vi "PXI-Set Property.vi"(0 "Key":string, 7 "Value":variant, 11 "error in (no error)":errorcluster) -> (15 "error out":errorcluster)   [LabVIEW 2015]
uses:
  DAQ Engine VIs/PXI Globals.vi
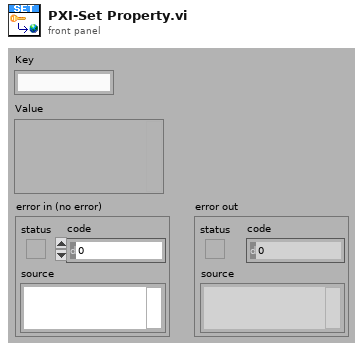
[diagram p1: front panel]
types:
  T1 = typedef "Counter Params.ctl" = cluster{"Counter":tag, "Hi ticks":u32, "Low ticks":u32, "Idle state":i32, "Delay ticks":u32}
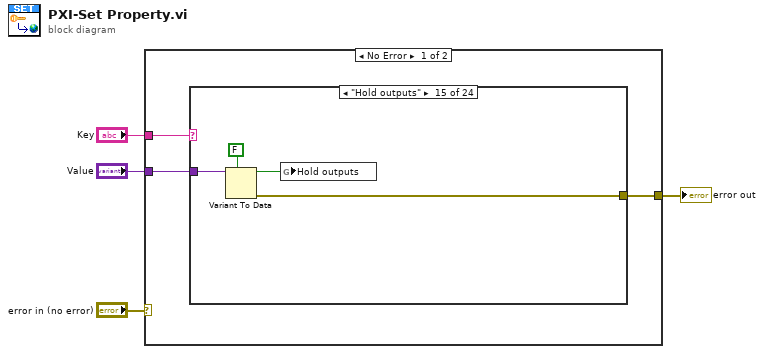
[diagram p0: block diagram]
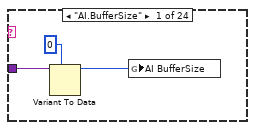
[diagram p2: hidden frame]
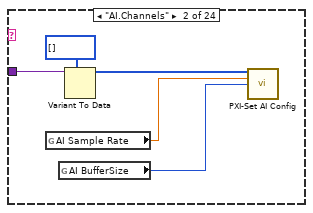
[diagram p3: hidden frame]
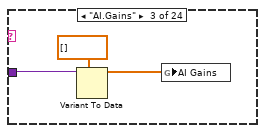
[diagram p4: hidden frame]
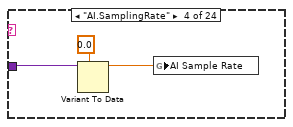
[diagram p5: hidden frame]
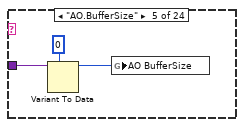
[diagram p6: hidden frame]
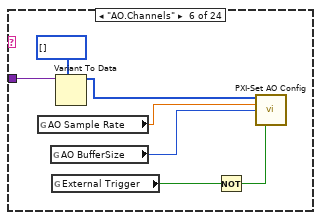
[diagram p7: hidden frame]
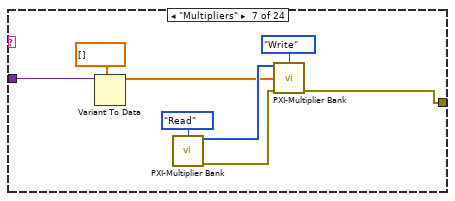
[diagram p8: hidden frame]
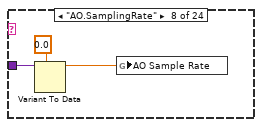
[diagram p9: hidden frame]
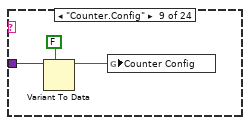
[diagram p10: hidden frame]
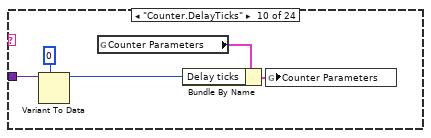
[diagram p11: hidden frame]
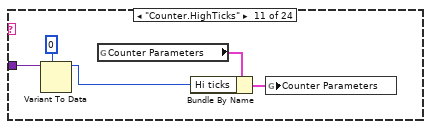
[diagram p12: hidden frame]
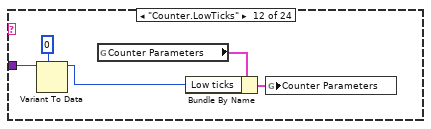
[diagram p13: hidden frame]
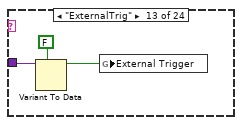
[diagram p14: hidden frame]
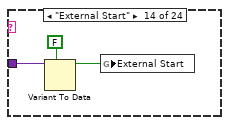
[diagram p15: hidden frame]
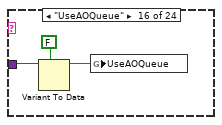
[diagram p16: hidden frame]
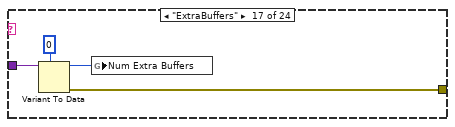
[diagram p17: hidden frame]
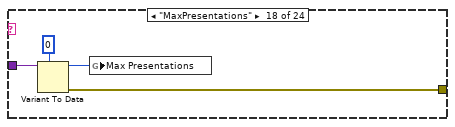
[diagram p18: hidden frame]
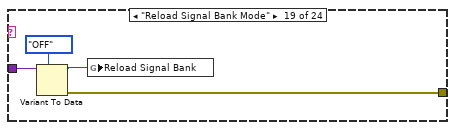
[diagram p19: hidden frame]
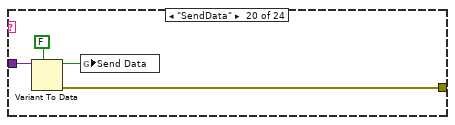
[diagram p20: hidden frame]
diagram:
  n1 = case shown="No Error" "error in (no error)" {
    selector: "error in (no error)" -> [_ w107]
    tunnel: "Key" -> [w7 _]
    tunnel: "Value" -> [w6 _]
    tunnel: [w5 w107] -> w1
    frame No Error {
      n2 = case shown="\"Hold outputs\"" w7 {
        selector: w7 -> [_ _ _ _ _ _ _ _ _ _ _ _ _ _ _ _ _ _ _ _ _ _ _ w104]
        tunnel: w6 -> [w10 w12 w17 w20 w23 w26 w33 w41 w44 w47 w52 w57 w62 w65 w69 w72 w76 w80 w85 w88 w92 w96 w100 _]
        tunnel: [_ _ _ _ _ _ w35 _ _ _ _ _ _ _ w67 _ w74 w78 w82 w86 w90 w94 w98 w102] -> w5
        frame "AI.BufferSize" {
          n3 = Variant To Data(type=0, Variant=w10) -> (data=w8:i32)  [unwired: 1 in, 1 out]
          n4 = global write "PXI Globals.vi" "AI BufferSize"(w8) -> ()
        }
        frame "AI.Channels" {
          n5 = global read "PXI Globals.vi" "AI Sample Rate"() -> (w15:dbl)
          n6 = global read "PXI Globals.vi" "AI BufferSize"() -> (w14:i32)
          n7 = Variant To Data(type=i32[] [], Variant=w12) -> (data=w11:i32[])  [unwired: 1 in, 1 out]
          n8 = call "PXI-Set AI Config.vi"("AI Channels"=w11, "Sampling Rate (Hz)"=w15, "Buffer Size"=w14) -> ()  [unwired: 12 in, 1 out]
        }
        frame "AI.Gains" {
          n9 = Variant To Data(type=dbl[] [], Variant=w17) -> (data=w16:dbl[])  [unwired: 1 in, 1 out]
          n10 = global write "PXI Globals.vi" "AI Gains"(w16) -> ()
        }
        frame "AI.SamplingRate" {
          n11 = Variant To Data(type=0.0, Variant=w20) -> (data=w19:dbl)  [unwired: 1 in, 1 out]
          n12 = global write "PXI Globals.vi" "AI Sample Rate"(w19) -> ()
        }
        frame "AO.BufferSize" {
          n13 = Variant To Data(type=0, Variant=w23) -> (data=w22:i32)  [unwired: 1 in, 1 out]
          n14 = global write "PXI Globals.vi" "AO BufferSize"(w22) -> ()
        }
        frame "AO.Channels" {
          n15 = global read "PXI Globals.vi" "AO Sample Rate"() -> (w31:dbl)
          n16 = global read "PXI Globals.vi" "AO BufferSize"() -> (w30:i32)
          n17 = global read "PXI Globals.vi" "External Trigger"() -> (w29:bool)
          n18 = Variant To Data(type=i32[] [], Variant=w26) -> (data=w25:i32[])  [unwired: 1 in, 1 out]
          n19 = Not(x=w29) -> (.not. x?=w28:bool)
          n20 = call "PXI-Set AO Config.vi"("AO Channels"=w25, "Sampling Rate (Hz)"=w31, "Buffer Size"=w30, "Regenerate"=w28) -> ()  [unwired: 11 in, 1 out]
        }
        frame "Multipliers" {
          n21 = Variant To Data(type=dbl[] [], Variant=w33) -> (data=w32:dbl[])  [unwired: 1 in, 1 out]
          n22 = call "PXI-Multiplier Bank.vi"("Action"=enum16{"Init", "Write", "Read"}."Read") -> ("Channels"=w37:i32[], "error out"=w36:errorcluster)  [unwired: 12 in, 1 out]
          n23 = call "PXI-Multiplier Bank.vi"("AO Channels"=w37, "Action"=enum16{"Init", "Write", "Read"}."Write", "Multipliers"=w32, "error in (no error)"=w36) -> ("error out"=w35:errorcluster)  [unwired: 9 in, 2 out]
        }
        frame "AO.SamplingRate" {
          n24 = Variant To Data(type=0.0, Variant=w41) -> (data=w40:dbl)  [unwired: 1 in, 1 out]
          n25 = global write "PXI Globals.vi" "AO Sample Rate"(w40) -> ()
        }
        frame "Counter.Config" {
          n26 = Variant To Data(type=FALSE, Variant=w44) -> (data=w43:bool)  [unwired: 1 in, 1 out]
          n27 = global write "PXI Globals.vi" "Counter Config"(w43) -> ()
        }
        frame "Counter.DelayTicks" {
          n28 = Variant To Data(type=0, Variant=w47) -> (data=w46:i32)  [unwired: 1 in, 1 out]
          n29 = global read "PXI Globals.vi" "Counter Parameters"() -> (w50:T1)
          n30 = Bundle By Name(cluster=w50, "Delay ticks"=w46) -> (w49:T1)
          n31 = global write "PXI Globals.vi" "Counter Parameters"(w49) -> ()
        }
        frame "Counter.HighTicks" {
          n32 = Variant To Data(type=0, Variant=w52) -> (data=w51:i32)  [unwired: 1 in, 1 out]
          n33 = global read "PXI Globals.vi" "Counter Parameters"() -> (w55:T1)
          n34 = Bundle By Name(cluster=w55, "Hi ticks"=w51) -> (w54:T1)
          n35 = global write "PXI Globals.vi" "Counter Parameters"(w54) -> ()
        }
        frame "Counter.LowTicks" {
          n36 = Variant To Data(type=0, Variant=w57) -> (data=w56:i32)  [unwired: 1 in, 1 out]
          n37 = global read "PXI Globals.vi" "Counter Parameters"() -> (w60:T1)
          n38 = Bundle By Name(cluster=w60, "Low ticks"=w56) -> (w59:T1)
          n39 = global write "PXI Globals.vi" "Counter Parameters"(w59) -> ()
        }
        frame "ExternalTrig" {
          n40 = Variant To Data(type=FALSE, Variant=w62) -> (data=w61:bool)  [unwired: 1 in, 1 out]
          n41 = global write "PXI Globals.vi" "External Trigger"(w61) -> ()
        }
        frame "External Start" {
          n42 = Variant To Data(type=FALSE, Variant=w65) -> (data=w64:bool)  [unwired: 1 in, 1 out]
          n43 = global write "PXI Globals.vi" "External Start"(w64) -> ()
        }
        frame "Hold outputs" {
          n44 = Variant To Data(type=FALSE, Variant=w69) -> (data=w68:bool, error out=w67:errorcluster)  [unwired: 1 in]
          n45 = global write "PXI Globals.vi" "Hold outputs"(w68) -> ()
        }
        frame "UseAOQueue" {
          n46 = Variant To Data(type=FALSE, Variant=w72) -> (data=w71:bool)  [unwired: 1 in, 1 out]
          n47 = global write "PXI Globals.vi" "UseAOQueue"(w71) -> ()
        }
        frame "ExtraBuffers" {
          n48 = Variant To Data(type=0, Variant=w76) -> (data=w75:i32, error out=w74:errorcluster)  [unwired: 1 in]
          n49 = global write "PXI Globals.vi" "Num Extra Buffers"(w75) -> ()
        }
        frame "MaxPresentations" {
          n50 = Variant To Data(type=0, Variant=w80) -> (data=w79:i32, error out=w78:errorcluster)  [unwired: 1 in]
          n51 = global write "PXI Globals.vi" "Max Presentations"(w79) -> ()
        }
        frame "Reload Signal Bank Mode" {
          n52 = Variant To Data(type=enum32{"OFF", "ENABLED", "FORCED"}."OFF" ("Reload Signal Bank"), Variant=w85) -> (data=w83:enum32{"OFF", "ENABLED", "FORCED"}, error out=w82:errorcluster)  [unwired: 1 in]
          n53 = global write "PXI Globals.vi" "Reload Signal Bank"(w83) -> ()
        }
        frame "SendData" {
          n54 = Variant To Data(type=FALSE, Variant=w88) -> (data=w87:bool, error out=w86:errorcluster)  [unwired: 1 in]
          n55 = global write "PXI Globals.vi" "Send Data"(w87) -> ()
        }
        frame "SkipSamples" {
          n56 = Variant To Data(type=0, Variant=w92) -> (data=w91:i32, error out=w90:errorcluster)  [unwired: 1 in]
          n57 = global write "PXI Globals.vi" "Skip Samples"(w91) -> ()
        }
        frame "Stop on MaxPresentations" {
          n58 = Variant To Data(type=FALSE, Variant=w96) -> (data=w95:bool, error out=w94:errorcluster)  [unwired: 1 in]
          n59 = global write "PXI Globals.vi" "Stop on MaxPresentations"(w95) -> ()
        }
        frame "TCPData" {
          n60 = Variant To Data(type=FALSE, Variant=w100) -> (data=w99:bool, error out=w98:errorcluster)  [unwired: 1 in]
          n61 = global write "PXI Globals.vi" "TCPData"(w99) -> ()
        }
        frame "ZZZ", Default {
          n62 = Format Into String(format string="Unexpected key: %s", w104) -> (resulting string=w103:string)  [unwired: 2 in, 1 out]
          n63 = call <vilib>:"Error Cluster From Error Code.vi"("error message (\"\")"=w103, "error code (0)"=-6000) -> ("error out"=w102:errorcluster)  [unwired: 7 in]
        }
      }
    }
    frame Error {
    }
  }
  "error out" <- w1
